vi "Set Initialization Data - AcquireWorker.vi"(8 "error in":errorcluster, 11 "ChartView Worker in":refnum<class "ChartView Worker.lvclass">) -> (0 "error out":errorcluster, 3 "ChartView Worker out":refnum<class "ChartView Worker.lvclass">)   [LabVIEW 2018, in "ChartView Worker.lvclass"]
doc: "Sets the initialization data of a statically linked subWorker."
uses:
  ChartView Worker.lvclass
  D:/Program Files (x86)/National Instruments/LabVIEW 2018/vi.lib/addons/_Workers/Library/Classes/Worker/Worker.lvclass
  Acquire Worker/Initialization Data.ctl
  <vilib>/addons/_Workers/Library/Classes/Message Queue/Message Queue.lvclass
  <vilib>/addons/_Workers/Library/Classes/Worker/Worker.lvclass/Worker.ctl
  ChartView Worker.lvclass/ChartView Worker.ctl
  Acquire Worker/DataAcquire Worker.lvclass
  <vilib>/addons/_Workers/Library/Classes/Worker/Worker.lvclass
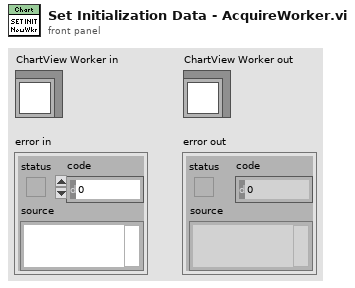
[diagram p1: front panel]
types:
  T1 = typedef "DataAcquire Worker.lvclass/Initialization Data.ctl" = cluster{"String":string, "Chart Queue":refnum<class "Message Queue.lvclass">}
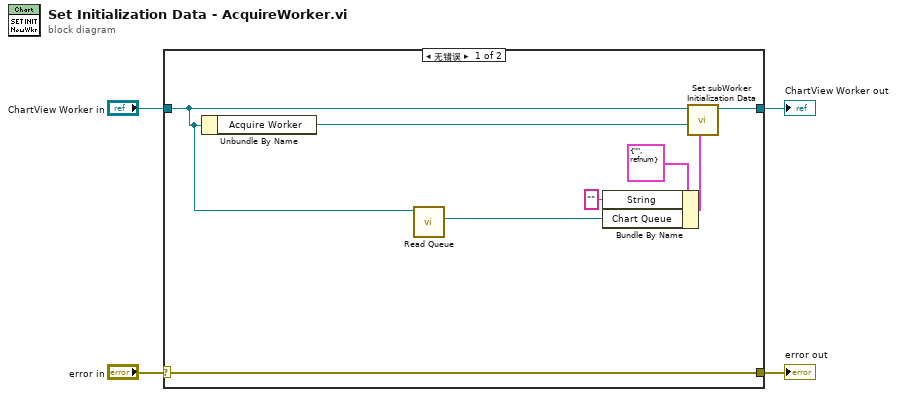
[diagram p0: block diagram]
diagram:
  n1 = case shown="无错误" "error in" {
    selector: "error in" -> [w12 w14]
    tunnel: [w12 w14] -> w3
    tunnel: [w11 w13] -> w2
    tunnel: "ChartView Worker in" -> [w5 w13]
    frame No Error {
      n2 = Unbundle By Name(w5) -> ("Acquire Worker"=w7:refnum<class "DataAcquire Worker.lvclass">)
      n3 = call <vilib>:"Read Queue.vi"("Worker"=w5) -> ("Message Queue out"=w6:refnum<class "Message Queue.lvclass">)  [unwired: 9 in, 1 out]
      n4 = Bundle By Name(cluster=T1 {"String"="", "Chart Queue"=refnum} ("Initialization Data"), "String"="" ("Placeholder"), "Chart Queue"=w6) -> (w9:T1)
      n5 = call-dynamic "Set subWorker Initialization Data.vi"("Initialization Data"=w9, "subWorker"=w7, "Worker"=w5) -> ("Worker out"=w11:refnum<class "ChartView Worker.lvclass">)  [unwired: 8 in]
    }
    frame Error {
    }
  }
  "error out" <- w3
  "ChartView Worker out" <- w2
